vi "Get Acquired Data.vi"(8 "error in (no error)":errorcluster, 11 "CCDCamera in":refnum<class "Simulated_CCD_Camera.lvclass">) -> (0 "error out":errorcluster, 3 "CCDCamera out":refnum<class "Simulated_CCD_Camera.lvclass">)   [LabVIEW 2018, in "Simulated_CCD_Camera.lvclass"]
uses:
  Simulated_CCD_Camera.lvclass
  Simulated_CCD_Camera.lvclass/Simulated_CCD_Camera.ctl
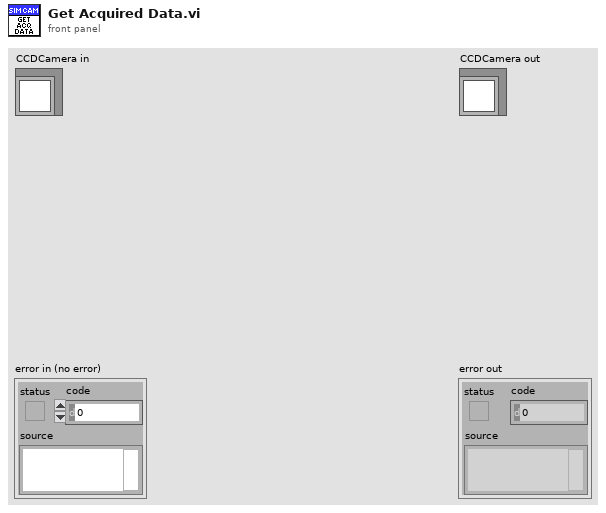
[diagram p1: front panel]
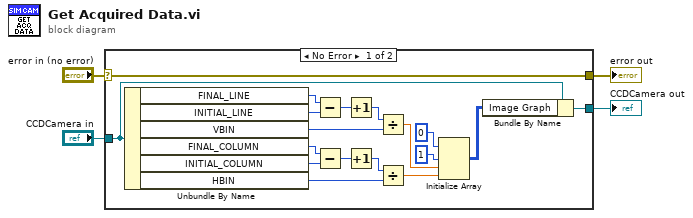
[diagram p0: block diagram]
diagram:
  n1 = case shown="No Error" "error in (no error)" {
    selector: "error in (no error)" -> [w11 w24]
    tunnel: [w11 w24] -> w1
    tunnel: [w22 w23] -> w2
    tunnel: "CCDCamera in" -> [w13 w23]
    frame No Error {
      n2 = Unbundle By Name(w13) -> ("FINAL_LINE"=w10:u16, "INITIAL_LINE"=w9:u16, "VBIN"=w8:u16, "FINAL_COLUMN"=w7:u16, "INITIAL_COLUMN"=w6:u16, "HBIN"=w5:u16)
      n3 = Subtract(x=w10, y=w9) -> (x-y=w21:u16)
      n4 = Subtract(x=w7, y=w6) -> (x-y=w20:u16)
      n5 = Increment(x=w21) -> (x+1=w19:u16)
      n6 = Increment(x=w20) -> (x+1=w18:u16)
      n7 = Divide(x=w19, y=w8) -> (x/y=w16:dbl)
      n8 = Divide(x=w18, y=w5) -> (x/y=w15:dbl)
      n9 = Initialize Array(u16 0, 1 ("dimension size"), w16, w15) -> (w14:u16[][][])
      n10 = Bundle By Name(cluster=w13, "Image Graph"=w14) -> (w22:refnum<class "Simulated_CCD_Camera.lvclass">)
    }
    frame Error {
    }
  }
  "error out" <- w1
  "CCDCamera out" <- w2
